vi "Desired Current to Voltage Command.vi"(11 "Desired Current":dbl) -> (3 "Voltage Command":dbl)   [LabVIEW 2018]
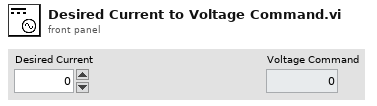
[diagram p1: front panel]
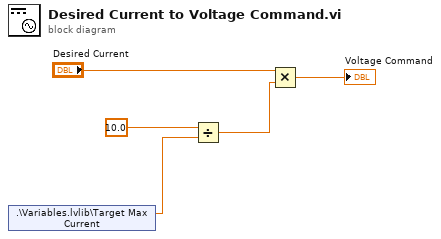
[diagram p0: block diagram]
diagram:
  n1 = shared-variable ".\\Variables.lvlib\\Target Max Current"() -> (w5:dbl)  [unwired: 1 in, 1 out]
  n2 = Divide(x=10.0, y=w5) -> (x/y=w2:dbl)
  n3 = Multiply(x="Desired Current", y=w2) -> (x*y=→"Voltage Command":dbl)
